vi "autonomus darrion style (WHS-ROB-6PZCBS1's conflicted copy 2013-02-20).vi"() -> ()   [LabVIEW 2010, in "Rampage.lvrbt"]
uses:
  Rampage.lvrbt
  <vilib>/NXT/Dual Mode Library/Waits/Wait_Num(msec).vi
  <vilib>/NXT/Subs/MotorOutput.ctl
  <vilib>/NXT/Subs/MotorXNode.DC Motor Type.ctl
  <vilib>/NXT/Subs/MotorXNode.2DCMotor.ctl
  <vilib>/NXT/Subs/LVHSConnector.ctl
  <vilib>/NXT/NXTIO Xnodes/NXTIONodeSubVIs/TETRIX IO Move DC Motors.vi
  <vilib>/NXT/NXTIO Xnodes/NXTIOXNode/NXTIO.xnode
  <vilib>/NXT/Dual Mode Library/Motors/MotorOn.vi
  <vilib>/NXT/Dual Mode Library/prims/inRangeAndCoerce/inRangeAndCoerce_int.vi
  <vilib>/NXT/NXTIO Xnodes/NXTIONodeSubVIs/TETRIX IO Stop DC Motors.vi
  <vilib>/NXT/NXTIO Xnodes/AddressXNode/NXTIOAddress.xnode
  <vilib>/NXT/Dual Mode Library/Waits/Wait_Num.vi
  <vilib>/NXT/Dual Mode Library/Sensors/Sonar_cm.vi
  <vilib>/NXT/Block Support/NXT_InputPort.ctl
panel:
  out "Enabled":bool
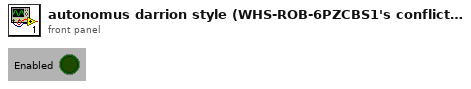
[diagram p1: front panel]
types:
  T1 = typedef "LVHSConnector.ctl" = cluster{"Hardware":string, "Flattened String":string}
  T2 = typedef "MotorOutput.ctl" = u8
  T3 = typedef "MotorXNode.DC Motor Type.ctl" = enum16{"DC Motor"}
  T4 = cluster{"DC Motor":T3, "Address":i16, "Address":i16}
  T5 = typedef "NXT_InputPort.ctl" = u8
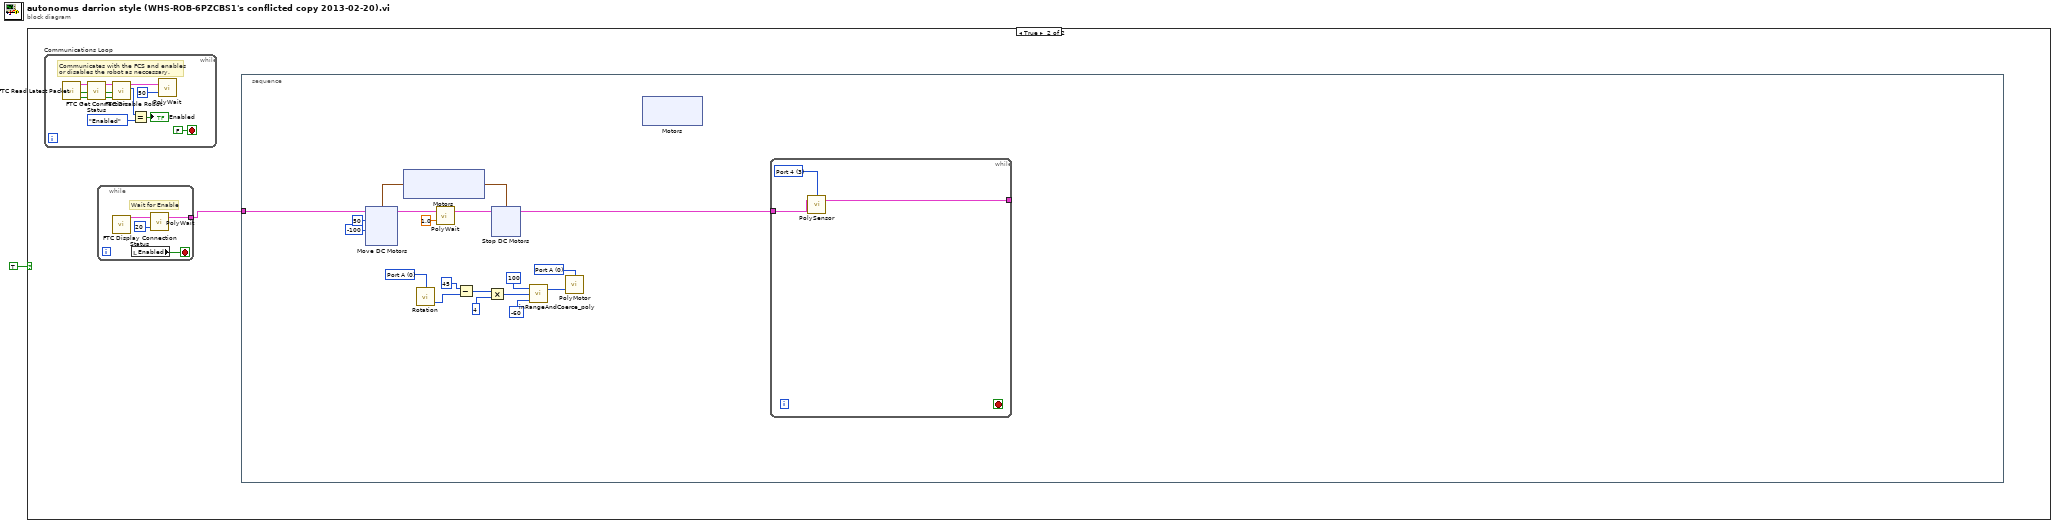
[diagram p0: block diagram]
diagram:
  n1 = case shown="True" TRUE {
    frame False {
    }
    frame True {
      n2 = while "Communications Loop" {
        stop <- FALSE stop-if-true
        # "Communicates with the FCS and enables \nor disables the robot as neccessary."
        n3 = call <vilib>:"FTC Read Latest Packet.vi"() -> ("Packet Received?"=w56:bool, "Stopped?"=w55:bool, "NXT"=w58:T1)  [unwired: 6 in, 3 out]
        n4 = call <vilib>:"FTC Get Connection Status.vi"("Packet Received?"=w56, "Stopped?"=w55, "NXT"=w58) -> ("Online?"=w47:bool, "Stopped?"=w48:bool, "NXT"=w57:T1)  [unwired: 5 in]
        n5 = call <vilib>:"FTC Disable Robot.vi"("Online?"=w47, "Stopped?"=w48, "NXT"=w57) -> ("Enabled?"=w51:enum16{"Disabled", "Enabled"}, "NXT"=w53:T1)  [unwired: 3 in]
        n6 = Equal?(x=w51, y=enum16{"Disabled", "Enabled"}."Enabled") -> (x = y?=→"Enabled":bool)
        n7 = call-poly <vilib>:"PolyWait.vi"("Time (100 msec)"=u32 50 ("Time (msec)"), "NXT"=w53) -> ()  [unwired: 2 in, 1 out]
      }
      n8 = while {
        tunnel: [w44] -> w2
        stop <- w45 stop-if-true
        # "Wait for Enable"
        n9 = call <vilib>:"FTC Display Connection Status.vi"() -> ("NXT"=w43:T1)  [unwired: 11 in]
        n10 = local read "Enabled"() -> (w45:bool)
        n11 = call-poly <vilib>:"PolyWait.vi"("Time (100 msec)"=u32 20 ("Time (msec)"), "NXT"=w43) -> ("NXT"=w44:T1)  [unwired: 2 in]
      }
      n12 = stacked-sequence {
        tunnel: w2 -> [w4]
        frame #0 {
          w12 = T2 0 items=["Port A"=0, "Port B"=1, "Port C"=2, "Ports A & B"=4, "Ports A & C"=5, "Ports B & C"=6, "All Ports"=3] ("Output Port (All Ports)")
          w10 = u8 0 items=["Port A", "Port B", "Port C"] ("Port (Port A)")
          n13 = xnode "Motors"() -> ("DC Motor"=w20:T4)
          n14 = xnode "Move DC Motors"("Power/Speed 1"=i8 50, "Motors"=w20, "NXT"=w4, "Power/Speed 2"=i8 -100) -> ("NXT"=w18:T1)
          n15 = call <vilib>:"Rotation.vi"("Port (Port A)"=w10) -> ("Angle of Rotation"=w13:i32)  [unwired: 2 in, 1 out]
          n16 = call-poly <vilib>:"PolyWait.vi"("Time (1 sec)"=sgl 1.0, "NXT"=w18) -> ("NXT"=w15:T1)  [unwired: 2 in]
          n17 = Subtract(x=45 ("Claw\nPosition"), y=w13) -> (x-y=w11:i32)
          n18 = Multiply(x=w11, y=4) -> (x*y=w9:i32)
          n19 = xnode "Stop DC Motors"("Motors"=w20, "NXT"=w15) -> ("NXT"=w3:T1)
          n20 = call-poly <vilib>:"inRangeAndCoerce_poly.vi"("lower limit"=-60, "x"=w9, "upper limit"=100) -> ("coerced(x)"=w6:i32)  [unwired: 1 out]
          n21 = call-poly <vilib>:"PolyMotor.vi"("Power (75)"=w6, "Output Port (All Ports)"=w12) -> ()  [unwired: 2 in, 1 out]
          n22 = xnode "Motors"() -> ()  [unwired: 1 out]
          n23 = while {
            tunnel: w3 -> [w23]
            tunnel: [w21] -> _
            stop <- _ stop-if-true
            w22 = T5 3 items=["Port 1", "Port 2", "Port 3", "Port 4"] ("Port (Port 4)")
            n24 = call-poly <vilib>:"PolySensor.vi"("NXT"=w23, "Port (Port 4)"=w22) -> ("NXT"=w21:T1)  [unwired: 1 in, 1 out]
          }
        }
      }
    }
  }
